vi "Init Max Size Data Array(2).vi"(9 "Data Stream Fmt Params":T1={"Samples per Block"=20, "Raw Data Status Len"=0, "Fltr Data Status Len"=0}, 10 "Max Samples":i32, 11 "Array Length":i32) -> (3 "initialized array":u32[][](array[numeric]))   [LabVIEW 2015, in "Tool Module.lvlib"]
uses:
  Tool Module.lvlib
  Tool Typedefs/_Data Stream Fmt Params Cluster--typedef.ctl
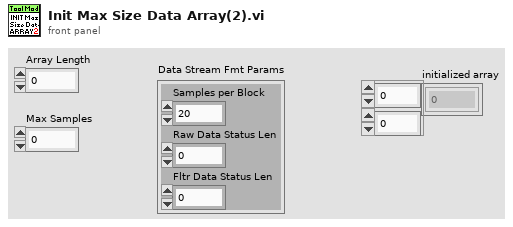
[diagram p1: front panel]
types:
  T1 = typedef "_Data Stream Fmt Params Cluster--typedef.ctl" = cluster{"Samples per Block":i32, "Raw Data Status Len":i32, "Fltr Data Status Len":i32}
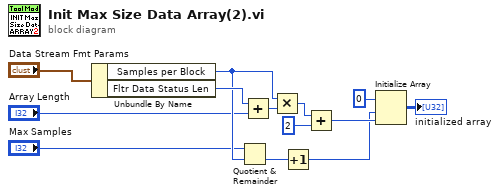
[diagram p0: block diagram]
diagram:
  n1 = Unbundle By Name("Data Stream Fmt Params") -> ("Samples per Block"=w4:i32, "Fltr Data Status Len"=w12:i32)
  n2 = Quotient & Remainder(x="Max Samples", y=w4) -> (floor(x/y)=w6:i32)  [unwired: 1 out]
  n3 = Add(x=w12, y="Array Length") -> (x+y=w11:i32)
  n4 = Multiply(x=w4, y=w11) -> (x*y=w10:i32)
  n5 = Increment(x=w6) -> (x+1=w5:i32)
  n6 = Add(x=w10, y=2) -> (x+y=w8:i32)
  n7 = Initialize Array(u32 0, w5, w8) -> (→"initialized array":u32[][])
